vi "Event Loop Processing.vi"(11 "Message Queue In":refnum<queue>) -> (0 "error out":errorcluster)   [LabVIEW 2023, in "HAF.lvlib" / "InteractionProcessor.lvclass"]
doc: "Manages events that can be received during processing and raises notifications for the main processing loop."
uses:
  InteractionProcessor.lvclass
  Message.ctl
  All Internal Message Ids.ctl
  Global Resources.vi
  HAF.lvlib
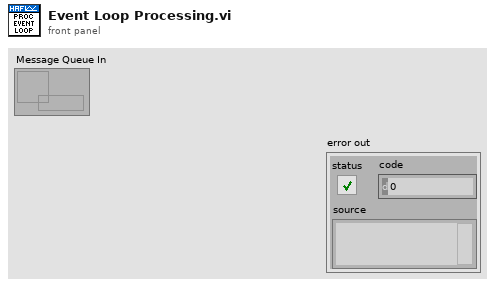
[diagram p1: front panel]
types:
  T1 = typedef "HAF.lvlib/All Events.ctl" = cluster{"Stop":T2, "Pause":T3, "Resume":T4, "Done":T5, "Injection":T6}
  T2 = typedef "HAF.lvlib/Stop Event.ctl" = refnum<user-event>
  T3 = typedef "HAF.lvlib/Pause Event.ctl" = refnum<user-event>
  T4 = typedef "HAF.lvlib/Resume Event.ctl" = refnum<user-event>
  T5 = typedef "HAF.lvlib/Done Event.ctl" = refnum<user-event>
  T6 = typedef "HAF.lvlib/Injection Event.ctl" = refnum<user-event>
  T7 = typedef "HAF.lvlib/All Internal Message Ids.ctl" = cluster{"Initialise":string, "Process":string, "Continue":string, "Done":string, "Pause":string, "Resume":string, "Stop":string, "Exit":string, "Inject":string}
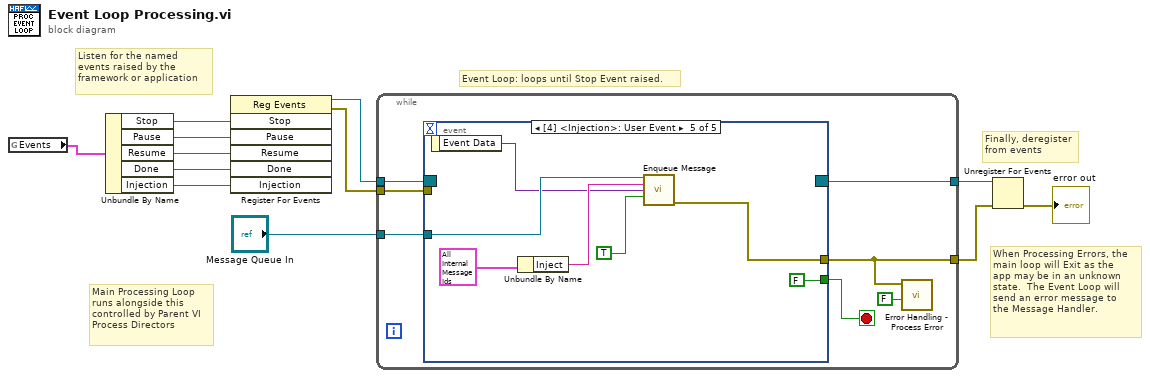
[diagram p0: block diagram]
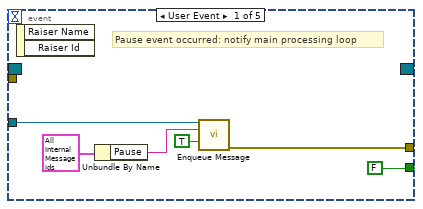
[diagram p2: hidden frame]
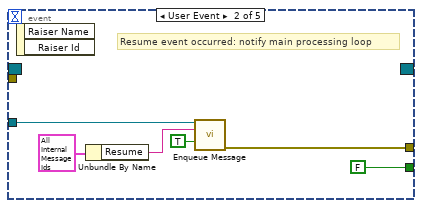
[diagram p3: hidden frame]
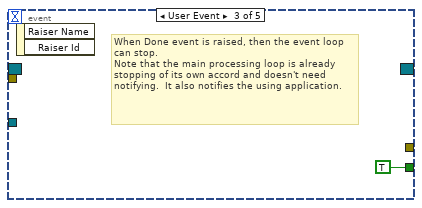
[diagram p4: hidden frame]
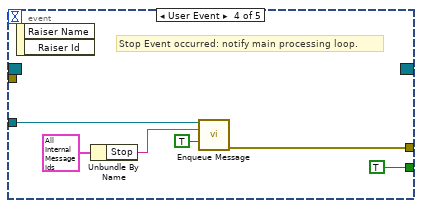
[diagram p5: hidden frame]
diagram:
  # "Main Processing Loop\nruns alongside this\ncontrolled by Parent VI\nProcess Directors"
  # "When Processing Errors, the\nmain loop will Exit as the\napp may be in an unknown\nstate.  The Event Loop will\nsend an error message to\nthe Message Handler."
  # "Finally, deregister\nfrom events"
  # "Listen for the named\nevents raised by the \nframework or application"
  # "Event Loop: loops until Stop Event raised."
  n1 = global read "Global Resources.vi" "Events"() -> (w12:T1)
  n2 = Unbundle By Name(w12) -> ("Stop"=w11:T2, "Pause"=w10:T3, "Resume"=w9:T4, "Done"=w8:T5, "Injection"=w1:T6)
  n3 = register-events(w11, w10, w9, w8, w1) -> (reference out=w7:refnum<event-registration>, error out=w6:errorcluster)  [unwired: 2 in]
  n4 = while {
    tunnel: w7 -> [w19]
    tunnel: w6 -> [w18]
    tunnel: "Message Queue In" -> [w17]
    tunnel: [w14] -> w3
    tunnel: [w15] -> w4
    stop <- w16 stop-if-true
    n5 = event shown="[4] <Injection>: User Event" {
      selector: w19 -> [_ _ _ _ _]
      dyn-events: [_ _ _ _ _] -> w15
      timeout: _ -> [_ _ _ _ _]
      tunnel: w18 -> [_ _ _ _ _]
      tunnel: w17 -> [w22 w28 _ w38 w43]
      tunnel: [w21 w27 _ w34 w42] -> w14
      tunnel: [FALSE FALSE TRUE TRUE FALSE] -> w16
      event User Event {
        # "Pause event occurred: notify main processing loop"
        n6 = event-data() -> ()  [unwired: 1 in, 2 out]
        n7 = Unbundle By Name(T7 {"Initialise"="Initialise", "Process"="Process", "Continue"="Continue", "Done"="Done", "Pause"="Pause", "Resume"="Resume", "Stop"="Stop", "Exit"="Exit", "Inject"=""} ("Message Ids")) -> ("Pause"=w25:string)
        n8 = call "Enqueue Message.vi"("Message Queue In"=w22, "Message Id"=w25, "Priority"=TRUE) -> ("error out"=w21:errorcluster)  [unwired: 11 in, 1 out]
      }
      event User Event {
        # "Resume event occurred: notify main processing loop"
        n9 = event-data() -> ()  [unwired: 1 in, 2 out]
        n10 = Unbundle By Name(T7 {"Initialise"="Initialise", "Process"="Process", "Continue"="Continue", "Done"="Done", "Pause"="Pause", "Resume"="Resume", "Stop"="Stop", "Exit"="Exit", "Inject"=""} ("Message Ids")) -> ("Resume"=w31:string)
        n11 = call "Enqueue Message.vi"("Message Queue In"=w28, "Message Id"=w31, "Priority"=TRUE) -> ("error out"=w27:errorcluster)  [unwired: 11 in, 1 out]
      }
      event User Event {
        # "When Done event is raised, then the event loop can stop.\nNote that the main processing loop is already stopping of its own accord and doesn't need notifying.  It also notifies the using application."
        n12 = event-data() -> ()  [unwired: 1 in, 2 out]
      }
      event User Event {
        # "Stop Event occurred: notify main processing loop."
        n13 = event-data() -> ()  [unwired: 1 in, 2 out]
        n14 = Unbundle By Name(T7 {"Initialise"="Initialise", "Process"="Process", "Continue"="Continue", "Done"="Done", "Pause"="Pause", "Resume"="Resume", "Stop"="Stop", "Exit"="Exit", "Inject"=""} ("Message Ids")) -> ("Stop"=w36:string)
        n15 = call "Enqueue Message.vi"("Message Queue In"=w38, "Message Id"=w36, "Priority"=TRUE) -> ("error out"=w34:errorcluster)  [unwired: 11 in, 1 out]
      }
      event User Event {
        n16 = event-data() -> ("Event Data"=w40:variant)  [unwired: 1 in]
        n17 = Unbundle By Name(T7 {"Initialise"="Initialise", "Process"="Process", "Continue"="Continue", "Done"="Done", "Pause"="Pause", "Resume"="Resume", "Stop"="Stop", "Exit"="Exit", "Inject"="Inject"} ("Message Ids")) -> ("Inject"=w45:string)
        n18 = call "Enqueue Message.vi"("Message Queue In"=w43, "Message Id"=w45, "Message Data"=w40, "Priority"=TRUE) -> ("error out"=w42:errorcluster)  [unwired: 10 in, 1 out]
      }
    }
    n19 = call "Error Handling - Process Error.vi"("Exit on Error"=FALSE, "error to process"=w14) -> ()  [unwired: 9 in, 1 out]
  }
  n20 = Unregister For Events(event registration refnum=w4, error in=w3) -> (error out=→"error out":errorcluster)
